vi "CAN Communication.vi"(7 "CAN Mode":T1, 8 "Error IN":errorcluster, 10 "Message":u8[](array[numeric]), 11 "Arbitration ID":u32) -> (0 "Error OUT":errorcluster)   [LabVIEW 2013]
uses:
  Type Defs/CAN Mode.ctl
  <vilib>/RioEmbeddedCAN/RioEmbeddedCAN.llb/CANFrameControl.ctl
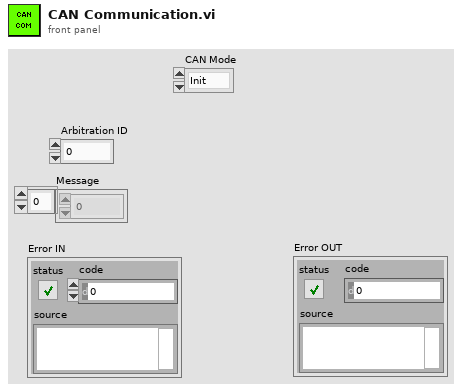
[diagram p1: front panel]
types:
  T1 = typedef "CAN Mode.ctl" = enum16{"Init", "Read", "Write", "Close"}
  T2 = typedef "CANFrameControl.ctl" = cluster{"identifier":u32, "extended?":bool, "type":enum8{"CAN Data", "CAN Remote"}, "payload":u8[]}
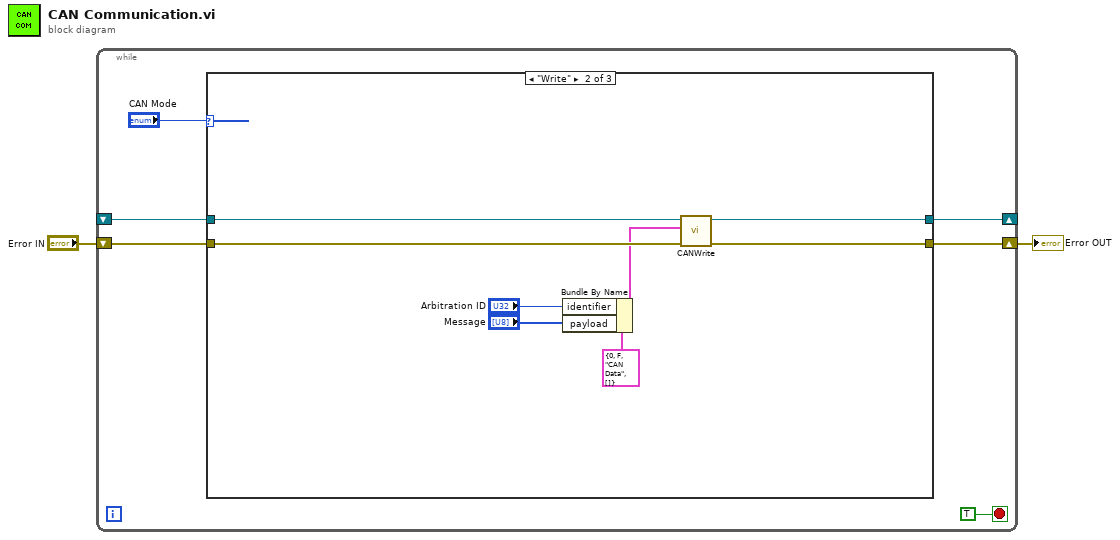
[diagram p0: block diagram]
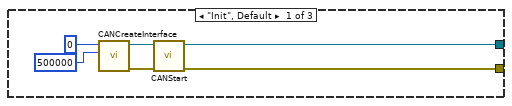
[diagram p2: hidden frame]
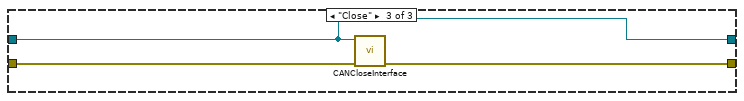
[diagram p3: hidden frame]
diagram:
  n1 = while {
    shift-right: [w6] -> _
    shift-left: _ -> [w4]
    shift-right: [w5] -> w1
    shift-left: "Error IN" -> [w3]
    stop <- TRUE stop-if-true
    n2 = case shown="\"Write\"" "CAN Mode" {
      tunnel: [w10 w20 w23] -> w6
      tunnel: [w9 w19 w24] -> w5
      tunnel: w4 -> [_ w22 w23]
      tunnel: w3 -> [_ w21 w25]
      frame "Init", Default {
        n3 = call <vilib>:"CANCreateInterface.vi"("baud rate"=u32 500000, "interface index"=u32 0) -> ("error out"=w11:errorcluster, "interface object out"=w12:refnum<k20>)  [unwired: 8 in]
        n4 = call <vilib>:"CANStart.vi"("error in (no error)"=w11, "interface object in"=w12) -> ("error out"=w9:errorcluster, "interface object out"=w10:refnum<k20>)  [unwired: 8 in]
      }
      frame "Write" {
        n5 = Bundle By Name(cluster=T2 {"identifier"=0, "extended?"=FALSE, "type"=enum."CAN Data", "payload"=[]} ("CAN frame"), "identifier"="Arbitration ID", "payload"="Message") -> (w17:T2)
        n6 = call <vilib>:"CANWrite.vi"("error in (no error)"=w21, "CAN frame"=w17, "interface object in"=w22) -> ("error out"=w19:errorcluster, "interface object out"=w20:refnum<k20>)  [unwired: 7 in]
      }
      frame "Close" {
        n7 = call <vilib>:"CANCloseInterface.vi"("error in (no error)"=w25, "interface object in"=w23) -> ("error out"=w24:errorcluster)  [unwired: 9 in]
      }
    }
  }
  "Error OUT" <- w1
